vi "Set Control Function.vi"(8 "error in":errorcluster, 9 "Function":T1, 10 "Device":T2) -> (0 "error out":errorcluster)   [LabVIEW 2024, in "FlexiFlowInterface.lvlib"]
doc: "Sets the control function.\n_____\nCreated using DQMH Event Scripter 7.0.1.1316."
uses:
  FlexiFlowInterface.lvlib
  FlexiFlowDevice--enum.ctl
  Modbus Flexi-Flow API/Control Function Values--enum.ctl
  Set Control Function Argument--cluster.ctl
  Modbus Flexi-Flow API/Bronkhorst Flexi-Flow ModbusTCP API.lvlib
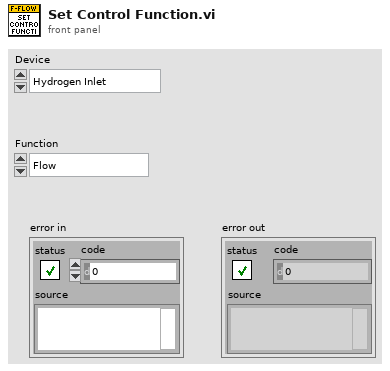
[diagram p1: front panel]
types:
  T1 = typedef "Bronkhorst Flexi-Flow ModbusTCP API.lvlib/Control Function Values--enum.ctl" = enum16{"Flow", "Upstream pressure", "Downstream pressure", "Flow with upstream pressure limit", "Flow with downstream pressure limit", "Upstream pressure with flow limit", "Downstream pressure with flow limit"}
  T2 = typedef "FlexiFlowInterface.lvlib/FlexiFlowDevice--enum.ctl" = enum16{"Hydrogen Inlet", "Nitrogen Inlet", "Cathode Outlet", "Anode Outlet"}
  T3 = typedef "FlexiFlowInterface.lvlib/Set Control Function Argument--cluster.ctl" = cluster{"Device":T2, "Function":T1}
  T4 = typedef "FlexiFlowInterface.lvlib/Request Events--cluster.ctl" = cluster{"Stop Module":refnum<user-event>, "Show Panel":refnum<user-event>, "Hide Panel":refnum<user-event>, "Get Module Execution Status":refnum<user-event>, "Show Diagram":refnum<user-event>, "Change Panel":refnum<user-event>, "Private":cluster{"Start Modbus Polling Helper Loop":refnum<user-event>, "Sleep Modbus Polling Helper Loop":refnum<user-event>, "Wake Connection Helper Loop":refnum<user-event>, "Sleep Connection Helper Loop":refnum<user-event>}, "Initialise Modbus Connections":refnum<user-event>, "Read Fmeasure":refnum<user-event>, "Set Modbus Configuration":refnum<user-event>, "Wink Devices":refnum<user-event>, "Read All FlexiFlow Device States":refnum<user-event>, "Wink Device":refnum<user-event>, "Set Control Function":refnum<user-event>, "Set Flow Setpoint":refnum<user-event>, "Set Backpressure Setpoint":refnum<user-event>, "Set Forward Pressure SP":refnum<user-event>, "Set Capacity Unit":refnum<user-event>, "Set Flow Capacity Unit":refnum<user-event>, "Set Setpoint Slope":refnum<user-event>, "Set Counter Settings":refnum<user-event>, "Reset All Device Counters":refnum<user-event>, "Read Device User Tag":refnum<user-event>, "Set Device User Tag":refnum<user-event>, "Read Counter Unit":refnum<user-event>, "Set Control Mode":refnum<user-event>, "Get Device Configuration":refnum<user-event>}
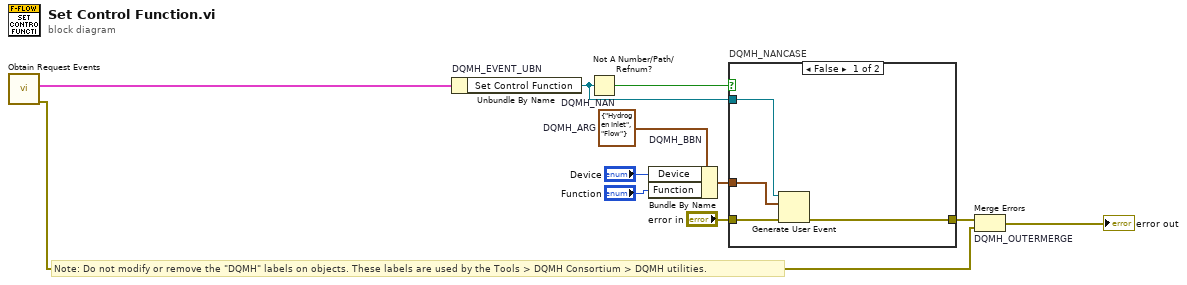
[diagram p0: block diagram]
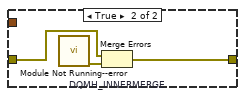
[diagram p2: hidden frame]
diagram:
  w5 = T3 {"Device"=enum."Hydrogen Inlet", "Function"=enum."Flow"}  # DQMH_ARG
  # "Note: Do not modify or remove the \"DQMH\" labels on objects. These labels are used by the Tools > DQMH Consortium > DQMH utilities."
  n1 = call "Obtain Request Events.vi"() -> ("error out"=w2:errorcluster, "FlexiFlowInterface Request Events"=w1:T4)  [unwired: 10 in]
  n2 = Unbundle By Name "DQMH_EVENT_UBN"(w1) -> ("Set Control Function"=w7:refnum<user-event>)
  n3 = Not A Number/Path/Refnum? "DQMH_NAN"(number/path/refnum=w7) -> (NaN/Path/Refnum?=w8:bool)
  n4 = Bundle By Name "DQMH_BBN"(cluster=w5, "Device"="Device", "Function"="Function") -> (w9:T3)
  n5 = case "DQMH_NANCASE" shown="False" w8 {
    tunnel: "error in" -> [w15 w18]
    tunnel: [w14 w17] -> w6
    tunnel: w7 -> [w13 _]
    tunnel: w9 -> [w12 _]
    frame False {
      n6 = Generate User Event(user event=w13, event data cluster=w12, error in=w15) -> (error out=w14:errorcluster)  [unwired: 1 in, 1 out]
    }
    frame True {
      n7 = call "Module Not Running--error.vi"() -> ("error out"=w16:errorcluster)  [unwired: 11 in]
      n8 = Merge Errors "DQMH_INNERMERGE"(w18, w16) -> (w17:errorcluster)
    }
  }
  n9 = Merge Errors "DQMH_OUTERMERGE"(w6, w2) -> (→"error out":errorcluster)
